vi "Build parameters unit test strings.vi"(9 "Expected":string, 10 "Value":string, 11 "Parameter":string) -> (3 "Chaîne 2":string)   [LabVIEW 2021]
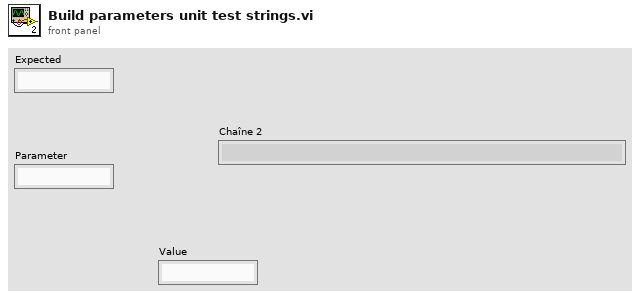
[diagram p1: front panel]
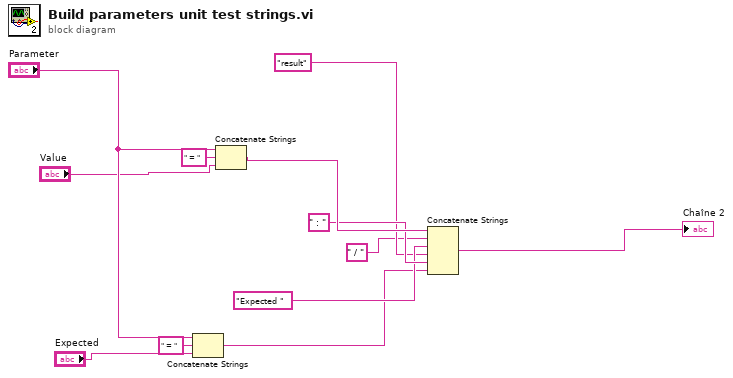
[diagram p0: block diagram]
diagram:
  n1 = Concatenate Strings("Parameter", " = " ("chaîne"), "Expected") -> (w1:string)
  n2 = Concatenate Strings("Parameter", " = " ("chaîne"), "Value") -> (w10:string)
  n3 = Concatenate Strings(w10, " / " ("chaîne"), "Expected " ("chaîne"), "result", " : " ("chaîne"), w1) -> (→"Chaîne 2":string)
